vi "Init_SetUP.vi"(8 "Error In":errorcluster) -> (0 "Error Out":errorcluster, 3 "Queue Cluster":T1)   [LabVIEW 2021, in "Queues.lvlib"]
doc: "This subVI is used to init the queue and user event of the SetUP VI."
uses:
  Queues.lvlib
  Tipski Definicii/SetUP_program_queues.ctl
  Tipski Definicii/Setup_sostojbi.ctl
panel:
  # "Input"
  # "Output"
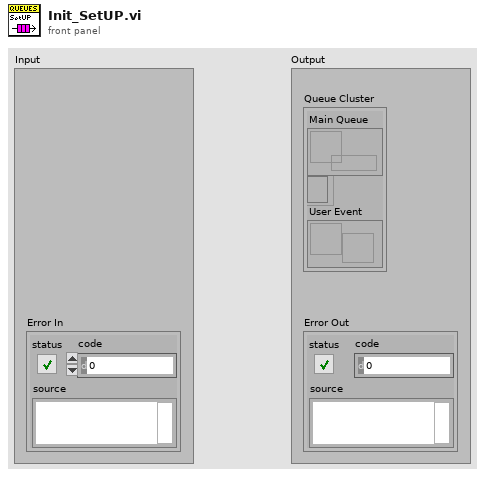
[diagram p1: front panel]
types:
  T1 = typedef "SetUP_program_queues.ctl" = cluster{"Main Queue":refnum<queue>, "ER Refnum":refnum<event-registration>, "User Event":refnum<user-event>}
  T2 = typedef "Setup_sostojbi.ctl" = enum16{"Init", "Generate Message ", "Setup", "End"}
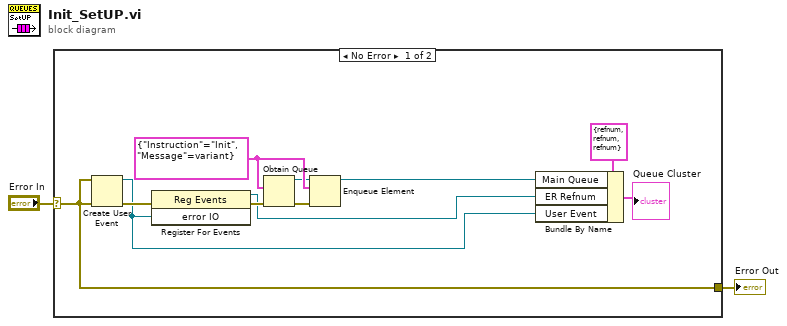
[diagram p0: block diagram]
diagram:
  n1 = case shown="No Error" "Error In" {
    selector: "Error In" -> [w3 w14]
    tunnel: [w3 w14] -> w1
    frame No Error {
      w13 = cluster{"Instruction":T2, "Message":variant} {"Instruction"=enum."Init", "Message"=variant}
      n2 = Create User Event(user event datatype=w3, error in=w3) -> (user event=w4:refnum<user-event>, error out=w9:errorcluster)
      n3 = register-events(error in=w9, w4) -> (reference out=w6:refnum<event-registration>, error out=w10:errorcluster)  [unwired: 1 in]
      n4 = Obtain Queue(element data type=w13, error in (no error)=w10) -> (queue out=w12:refnum<queue>, error out=w11:errorcluster)  [unwired: 3 in, 1 out]
      n5 = Enqueue Element(queue=w12, element=w13, error in (no error)=w11) -> (queue out=w7:refnum<queue>)  [unwired: 1 in, 2 out]
      n6 = Bundle By Name(cluster=T1 {"Main Queue"=refnum, "ER Refnum"=refnum, "User Event"=refnum}, "Main Queue"=w7, "ER Refnum"=w6, "User Event"=w4) -> (→"Queue Cluster":T1)
    }
    frame Error {
    }
  }
  "Error Out" <- w1
